vi "LVClass_Pupil dtor.vi"(0 "Pupil in":refnum<class "Pupil.lvclass">, 11 "error in (no error)":errorcluster) -> (4 "Pupil out":refnum<class "Pupil.lvclass">, 15 "error out":errorcluster)   [LabVIEW 2020, in "Pupil.lvclass"]
doc: "Pupil destructor.\n\n--------------------------------------------------------------------------------\n\n<B>PupilIn </B> : Pupil object.\n<B>PupilOut </B> : Pupil object.\n<B>ErrorIn </B> : Error\n<B>ErrorOut </B> : Error\n\n--------------------------------------------------------------------------------"
uses:
  Pupil.lvclass
  Pupil.lvclass/Pupil.ctl
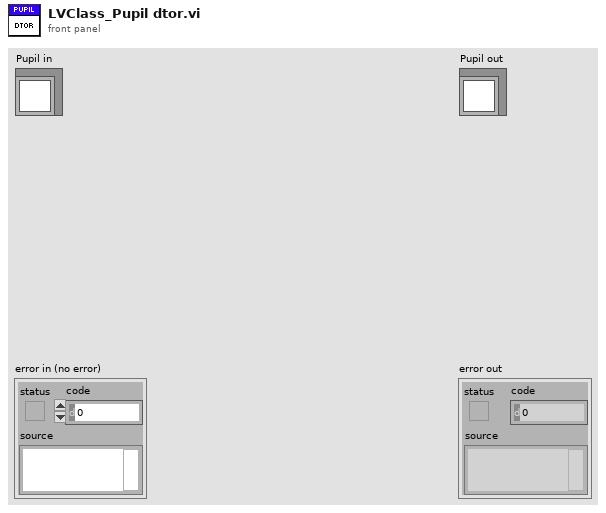
[diagram p1: front panel]
types:
  T1 = typedef "Handle creation.ctl" = enum16{"By ctor", "By write function"}
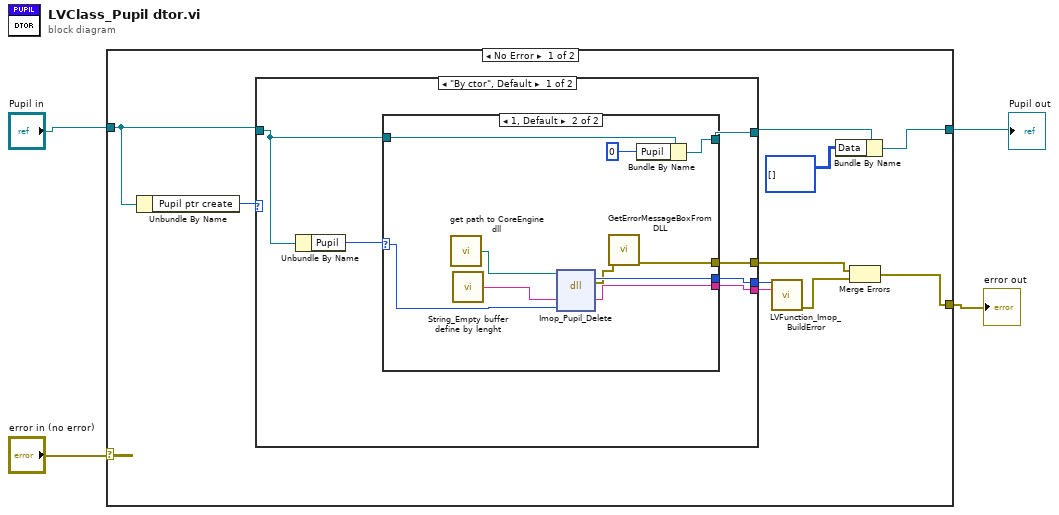
[diagram p0: block diagram]
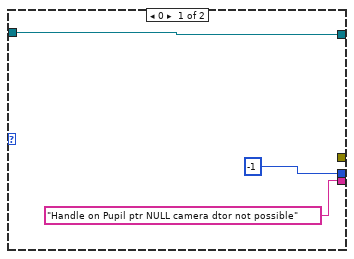
[diagram p2: hidden frame]
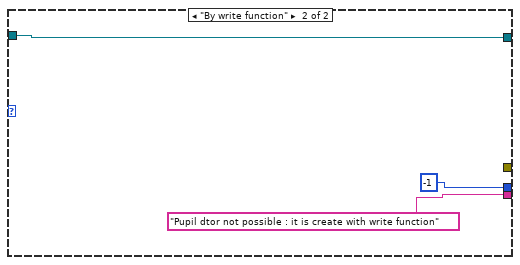
[diagram p3: hidden frame]
diagram:
  n1 = case shown="No Error" "error in (no error)" {
    selector: "error in (no error)" -> [_ w37]
    tunnel: "Pupil in" -> [w12 w38]
    tunnel: [w6 w38] -> w1
    tunnel: [w9 w37] -> w2
    frame No Error {
      n2 = Unbundle By Name(w12) -> ("Pupil ptr create"=w11:T1)
      n3 = case shown="\"By ctor\", Default" w11 {
        tunnel: [w20 "Pupil dtor not possible : it is create with write function" ("message")] -> w14
        tunnel: [w19 -1] -> w13
        tunnel: w12 -> [w17 w36]
        tunnel: [w18 w36] -> w7
        tunnel: [w15 _] -> w8
        frame "By ctor", Default {
          n4 = Unbundle By Name(w17) -> ("Pupil"=w16:i32)
          n5 = case shown="1, Default" w16 {
            selector: w16 -> [_ w30]
            tunnel: ["Handle on Pupil ptr NULL camera dtor not possible" ("message") w32] -> w20
            tunnel: [-1 w31] -> w19
            tunnel: w17 -> [w21 w26]
            tunnel: [w21 w25] -> w18
            tunnel: [_ w24] -> w15
            frame 0 {
            }
            frame 1, Default {
              n6 = call "get path to CoreEngine dll.vi"() -> ("path to c_interface_vc100.dll"=w29:path)  [unwired: 12 in, 3 out]
              n7 = call "String_Empty buffer define by lenght.vi"() -> ("Empty buffer"=w33:string)  [unwired: 1 in]
              n8 = dll-call lib="D:/soft/HASO_v3/SVN_trunk/ImOpCoreEngine4_LV2011/DLLs/c_interface_vc100.dll" fn="Imop_Pupil_Delete"(path in=w29, "message"=w33, "objet"=w30) -> (error out=w28:errorcluster, "return type"=w31:i32, "message"=w32:string)  [unwired: 3 in, 1 out]
              n9 = call "GetErrorMessageBoxFromDLL.vi"("error IN"=w28) -> ("error OUT"=w24:errorcluster)  [unwired: 10 in]
              n10 = Bundle By Name(cluster=w26, "Pupil"=u32 0) -> (w25:refnum<class "Pupil.lvclass">)
            }
          }
        }
        frame "By write function" {
        }
      }
      n11 = call "LVFunction_Imop_BuildError.vi"("code"=w13, "String to Prepend to source (\"\")"=w14) -> ("error out"=w10:errorcluster)  [unwired: 13 in]
      n12 = Bundle By Name(cluster=w7, "Data"=i32[][] []) -> (w6:refnum<class "Pupil.lvclass">)
      n13 = Merge Errors(w8, w10) -> (w9:errorcluster)
    }
    frame Error {
    }
  }
  "error out" <- w2
  "Pupil out" <- w1
